vi "DispatchService wrapper.vi"(8 "error in (no error)":errorcluster, 9 "Dispatch Service? (f)":bool) -> (0 "error out":errorcluster)   [LabVIEW 2011]
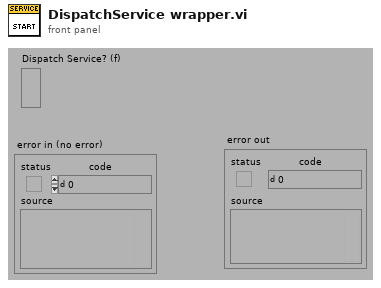
[diagram p1: front panel]
types:
  T1 = typedef "Rendezvous RefNum" = refnum<k1>
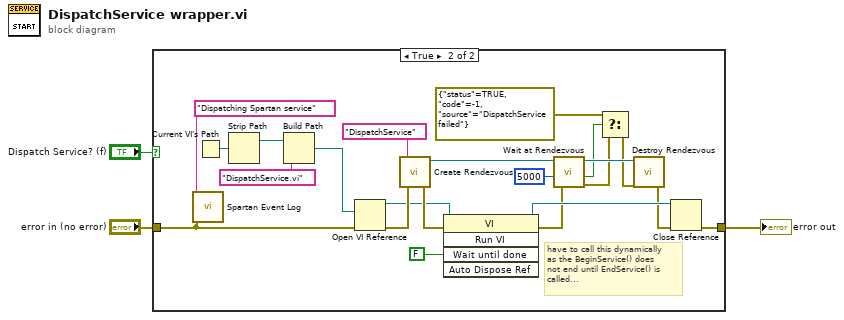
[diagram p0: block diagram]
diagram:
  n1 = case shown="True" "Dispatch Service? (f)" {
    tunnel: "error in (no error)" -> [w4 w18]
    tunnel: [w4 w21] -> w1
    frame False {
    }
    frame True {
      # "have to call this dynamically\nas the BeginService() does\nnot end until EndService() is\ncalled..."
      n2 = call "Spartan Event Log.vi"("error in (no error)"=w18, "message (\"\")"="Dispatching Spartan service") -> ()  [unwired: 3 in, 4 out]
      n3 = Current VI's Path() -> (path=w25:path)
      n4 = Strip Path(path=w25) -> (stripped path=w24:path)  [unwired: 1 out]
      n5 = Build Path(base path=w24, name or relative path="DispatchService.vi") -> (appended path=w22:path)
      n6 = Open VI Reference(vi path=w22, error in (no error)=w18) -> (vi reference=w5:refnum<vi>, error out=w17:errorcluster)  [unwired: 4 out]
      n7 = call <vilib>:"Create Rendezvous.vi"("error in (no error)"=w17, "name (unnamed)"="DispatchService") -> ("error out"=w6:errorcluster, "rendezvous"=w15:T1)  [unwired: 3 in, 1 out]
      n8 = invoke class="VI" method="Run VI"(reference=w5, error in=w6, "Wait until done"=FALSE) -> (reference out=w20:refnum<vi>, error out=w13:errorcluster)  [unwired: 2 in, 3 out]
      n9 = call <vilib>:"Wait at Rendezvous.vi"("error in (no error)"=w13, "ms timeout (-1)"=5000, "rendezvous"=w15) -> ("error out"=w9:errorcluster, "timed out"=w10:bool, "rendezvous out"=w14:T1)  [unwired: 2 in]
      n10 = Select(t=errorcluster {"status"=TRUE, "code"=-1, "source"="DispatchService failed"}, s=w10, f=w9) -> (s? t:f=w8:errorcluster)
      n11 = call <vilib>:"Destroy Rendezvous.vi"("error in (no error)"=w8, "rendezvous"=w14) -> ("error out"=w12:errorcluster)  [unwired: 4 in, 1 out]
      n12 = Close Reference(reference=w20, error in (no error)=w12) -> (error out=w21:errorcluster)
    }
  }
  "error out" <- w1
